vi "Read TypeFirmware.vi"(8 "error in (no error)":errorcluster, 11 "XuLyStringUART in":refnum<class "XuLyStringUART.lvclass">) -> (0 "error out":errorcluster, 2 "TypeFirmware":T1, 3 "XuLyStringUART out":refnum<class "XuLyStringUART.lvclass">)   [LabVIEW 2017, in "LibraryGcode.lvlib" / "XuLyStringUART.lvclass"]
uses:
  XuLyStringUART.lvclass
  control/TypeFirmwareControl.ctl
  XuLyStringUART.lvclass/XuLyStringUART.ctl
  LibraryGcode.lvlib
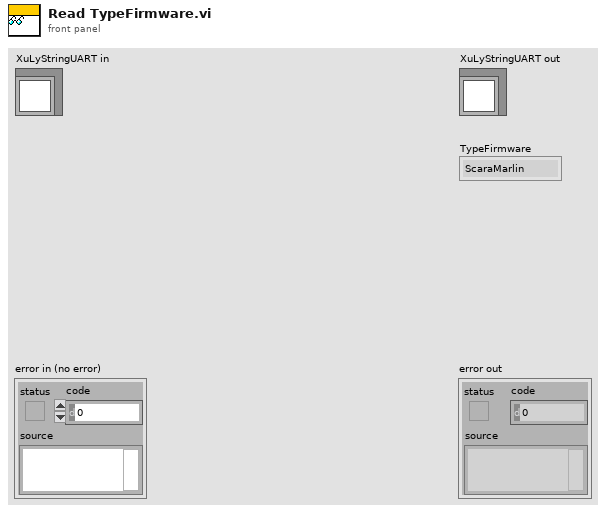
[diagram p1: front panel]
types:
  T1 = typedef "LibraryGcode.lvlib/TypeFirmwareControl.ctl" = enum16{"ScaraMarlin", "CncMarlin", "Mk4Due"}
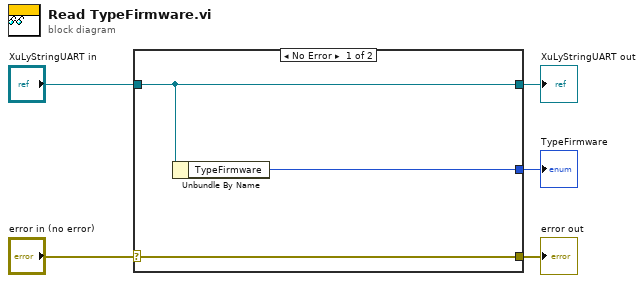
[diagram p0: block diagram]
diagram:
  n1 = case shown="No Error" "error in (no error)" {
    selector: "error in (no error)" -> [w8 w9]
    tunnel: [w8 w9] -> w4
    tunnel: [w7 w10] -> w2
    tunnel: "XuLyStringUART in" -> [w7 w10]
    tunnel: [w6 _] -> w1
    frame No Error {
      n2 = Unbundle By Name(w7) -> ("TypeFirmware"=w6:T1)
    }
    frame Error {
    }
  }
  "error out" <- w4
  "XuLyStringUART out" <- w2
  "TypeFirmware" <- w1
